vi "队列.vi"() -> ()   [LabVIEW 2019]
panel:
  in  "队列输出 3":refnum<queue>
  in  "队列输出 2":refnum<queue>
  in  "队列输出":refnum<queue>
  in  "停止":bool
  out "元素":i32
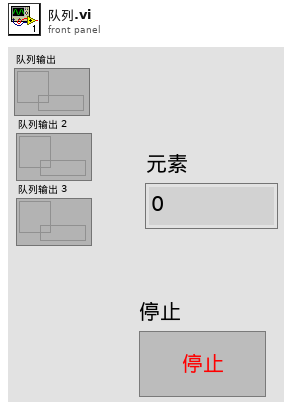
[diagram p1: front panel]
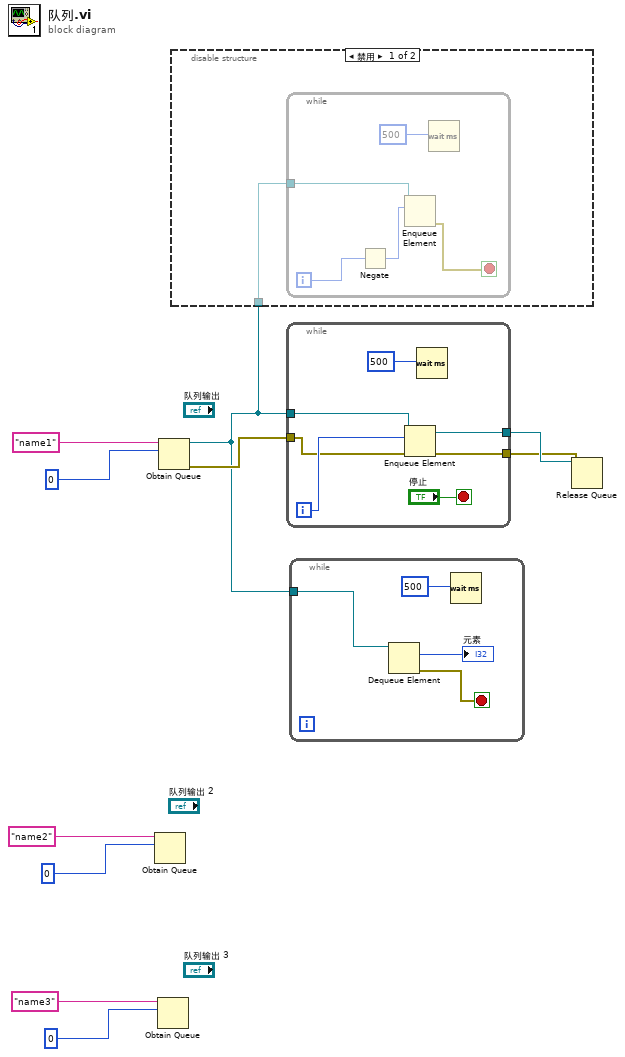
[diagram p0: block diagram]
diagram:
  n1 = Obtain Queue(name (unnamed)="name2" ("名称（未命名）"), element data type=0) -> ()  [unwired: 3 in, 3 out]
  n2 = Obtain Queue(name (unnamed)="name3" ("名称（未命名）"), element data type=0) -> ()  [unwired: 3 in, 3 out]
  n3 = Obtain Queue(name (unnamed)="name1" ("名称（未命名）"), element data type=0) -> (queue out=w5:refnum<queue>, error out=w10:errorcluster)  [unwired: 3 in, 1 out]
  n4 = disable-structure shown="禁用" {
    disable-tunnel: w5 -> [w11 _]
    frame Disabled {
      n5 = while {
        tunnel: w11 -> [w16]
        i -> [w15]
        stop <- w13 stop-if-true
        n6 = Negate(x=w15) -> (-x=w14:i32)
        n7 = Enqueue Element(queue=w16, element=w14) -> (error out=w13:errorcluster)  [unwired: 2 in, 2 out]
        n8 = Wait (ms)(milliseconds to wait=u32 500 ("毫秒计时值")) -> ()  [unwired: 1 out]
      }
    }
    frame Enabled {
    }
  }
  n9 = while {
    tunnel: w5 -> [w23]
    tunnel: w10 -> [w18]
    tunnel: [w21] -> w7
    tunnel: [w20] -> w6
    i -> [w22]
    stop <- "停止" stop-if-true
    n10 = Enqueue Element(queue=w23, element=w22, error in (no error)=w18) -> (queue out=w21:refnum<queue>, error out=w20:errorcluster)  [unwired: 1 in, 1 out]
    n11 = Wait (ms)(milliseconds to wait=u32 500 ("毫秒计时值")) -> ()  [unwired: 1 out]
  }
  n12 = while {
    tunnel: w5 -> [w27]
    stop <- w26 stop-if-true
    n13 = Dequeue Element(queue=w27) -> (element=→"元素":i32, error out=w26:errorcluster)  [unwired: 2 in, 2 out]
    n14 = Wait (ms)(milliseconds to wait=u32 500 ("毫秒计时值")) -> ()  [unwired: 1 out]
  }
  n15 = Release Queue(queue=w7, error in (no error)=w6) -> ()  [unwired: 1 in, 3 out]
